vi "Parse Bits.vi"(8 "error in (no error)":errorcluster, 11 "Operator in":refnum<class "Operator.lvclass">) -> (0 "error out":errorcluster, 3 "Operator out":refnum<class "Operator.lvclass">)   [LabVIEW 2020, in "Operator.lvclass"]
uses:
  Operator.lvclass
  C:/dev/IlluminatedG/AdventOfCode/2021/source/Day 16/Part 1/Packet/Packet.lvclass
  Operator.lvclass/Operator.ctl
  Packet/Packet.lvclass
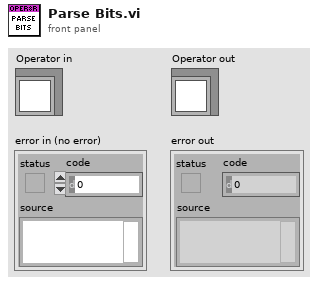
[diagram p1: front panel]
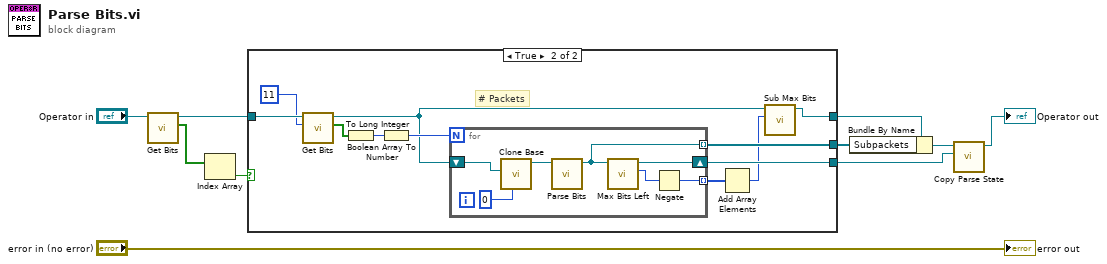
[diagram p0: block diagram]
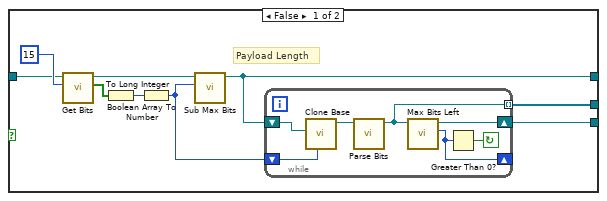
[diagram p2: hidden frame]
diagram:
  n1 = call "Get Bits.vi"("Packet in"="Operator in") -> ("Bits"=w8:bool[], "Packet out"=w1:refnum<class "Operator.lvclass">)  [unwired: 8 in, 1 out]
  n2 = Index Array(array=w8) -> (element=w7:bool)  [unwired: 1 in]
  n3 = case shown="True" w7 {
    tunnel: w1 -> [w14 w33]
    tunnel: [w11 w28] -> w6
    tunnel: [w19 w37] -> w5
    tunnel: [w18 w36] -> w3
    frame False {
      # "Payload Length"
      n4 = call "Get Bits.vi"("Count (1)"=15, "Packet in"=w14) -> ("Bits"=w16:bool[], "Packet out"=w13:refnum<class "Operator.lvclass">)  [unwired: 7 in, 1 out]
      n5 = Boolean Array To Number(Boolean array=w16) -> (number=w17:u32)
      n6 = To Long Integer(number=w17) -> (32bit integer=w12:i32)
      n7 = call "Sub Max Bits.vi"("Count"=w12, "Packet in"=w13) -> ("Packet out"=w11:refnum<class "Operator.lvclass">)  [unwired: 8 in, 1 out]
      n8 = while {
        shift-right: [w22] -> w18
        shift-left: w11 -> [w25]
        shift-right: [w21] -> _
        shift-left: w12 -> [w20]
        tunnel: [w23] -> w19 mode=indexing
        stop <- w26 continue-if-true
        n9 = call "Clone Base.vi"("Max Bits"=w20, "From"=w25) -> ("Packet in"=w24:refnum<class "Packet.lvclass">)  [unwired: 8 in, 1 out]
        n10 = call-dynamic "Parse Bits.vi"("Packet in"=w24) -> ("Packet out"=w23:refnum<class "Packet.lvclass">)  [unwired: 9 in, 1 out]
        n11 = call "Max Bits Left.vi"("Packet in"=w23) -> ("Max Bits Left"=w21:i32, "Packet out"=w22:refnum<class "Packet.lvclass">)  [unwired: 8 in, 1 out]
        n12 = Greater Than 0?(x=w21) -> (x > 0?=w26:bool)
      }
    }
    frame True {
      # "# Packets"
      n13 = call "Get Bits.vi"("Count (1)"=11, "Packet in"=w33) -> ("Bits"=w34:bool[], "Packet out"=w29:refnum<class "Operator.lvclass">)  [unwired: 7 in, 1 out]
      n14 = Boolean Array To Number(Boolean array=w34) -> (number=w35:u32)
      n15 = To Long Integer(number=w35) -> (32bit integer=w32:i32)
      n16 = for {
        N: w32 -> [_]
        shift-right: [w42] -> w36
        shift-left: w29 -> [w44]
        tunnel: [w41] -> w37 mode=indexing
        tunnel: [w39] -> w30 mode=indexing
        n17 = call "Clone Base.vi"("Max Bits"=0, "From"=w44) -> ("Packet in"=w43:refnum<class "Packet.lvclass">)  [unwired: 8 in, 1 out]
        n18 = call-dynamic "Parse Bits.vi"("Packet in"=w43) -> ("Packet out"=w41:refnum<class "Packet.lvclass">)  [unwired: 9 in, 1 out]
        n19 = call "Max Bits Left.vi"("Packet in"=w41) -> ("Max Bits Left"=w40:i32, "Packet out"=w42:refnum<class "Packet.lvclass">)  [unwired: 8 in, 1 out]
        n20 = Negate(x=w40) -> (-x=w39:i32)
      }
      n21 = Add Array Elements(numeric array=w30) -> (sum=w27:i32)
      n22 = call "Sub Max Bits.vi"("Count"=w27, "Packet in"=w29) -> ("Packet out"=w28:refnum<class "Operator.lvclass">)  [unwired: 8 in, 1 out]
    }
  }
  n23 = Bundle By Name(cluster=w6, "Subpackets"=w5) -> (w4:refnum<class "Operator.lvclass">)
  n24 = call "Copy Parse State.vi"("From"=w3, "Packet in"=w4) -> ("Packet out"=→"Operator out":refnum<class "Operator.lvclass">)  [unwired: 8 in, 1 out]
  "error out" <- "error in (no error)"
